vi "getDescription.vi"(8 "error in (no error)":errorcluster, 11 "Xcite in":refnum<class "Xcite.lvclass">) -> (0 "error out":errorcluster, 2 "description":T1={"serial"=0, "type"=65535, "name"="", "wavelenghts_vec"=[], "exclusivity_vec"=[], "intensity_max_vec"=[], "intensity_min_vec"=[]} {"type" items=["XC_120PC"=0, "XC_exacte"=1, "XC_120LED"=2, "XC_110LED"=3, "XC_mini"=4, "XC_XYLIS"=5, "XC_XR210"=6, "XC_LED1"=7, "XC_XT600"=8, "XC_XT900"=9, "Any"=65535]}, 3 "Xcite out":refnum<class "Xcite.lvclass">)   [LabVIEW 2019, in "Xcite.lvclass"]
doc: "Gets the serial number, type and other properties of the XCite device"
uses:
  Xcite.lvclass
  Xcite.lvclass/Xcite.ctl
  etc.xcite/XCite.lvlib
panel:
  out "XCiteType":u16(ring) format="%x" items=["XC_120PC"=0, "XC_exacte"=1, "XC_120LED"=2, "XC_110LED"=3, "XC_mini"=4, "XC_XYLIS"=5, "XC_XR210"=6, "XC_LED1"=7, "XC_XT600"=8, "XC_XT900"=9, "Any"=65535]
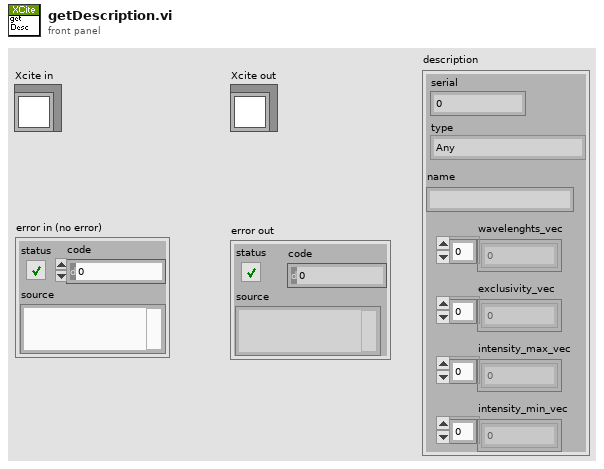
[diagram p1: front panel]
types:
  T1 = cluster{"serial":u32, "type":u16, "name":string, "wavelenghts_vec":u32[], "exclusivity_vec":u32[], "intensity_max_vec":u32[], "intensity_min_vec":u32[]}
  T2 = cluster{"LightSourceName":string, "hDevice":u64, "hCamera":u64, "iNumChannels":i32, "iNumWheels":i32, "dwSystemState":u32, "dwSerialNumber":u32, "dwSystemCaps":u32, "iLastChannelOnWheel":i16[], "XCiteChannels":cluster{"szLedName":string, "iWaveLength":i32, "IBelongToWheelNumber":i32, "iIntensity":i32, "iIntensityMin":i32, "iIntensityMax":i32, "iIntensityStep":i32, "iExtTriggerNum":i32, "iLedTemp":i32, "dwLEDState":u32}[]}
  T3 = cluster{"szLedName":string, "iWaveLength":i32, "IBelongToWheelNumber":i32, "iIntensity":i32, "iIntensityMin":i32, "iIntensityMax":i32, "iIntensityStep":i32, "iExtTriggerNum":i32, "iLedTemp":i32, "dwLEDState":u32}[]
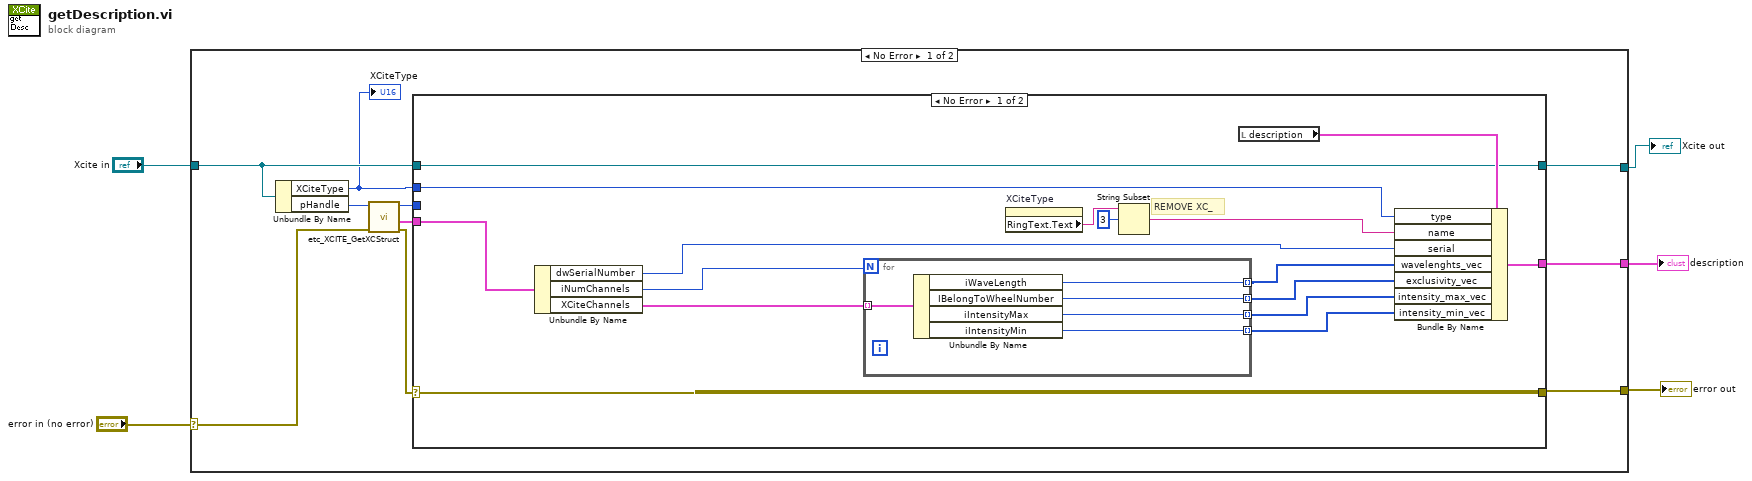
[diagram p0: block diagram]
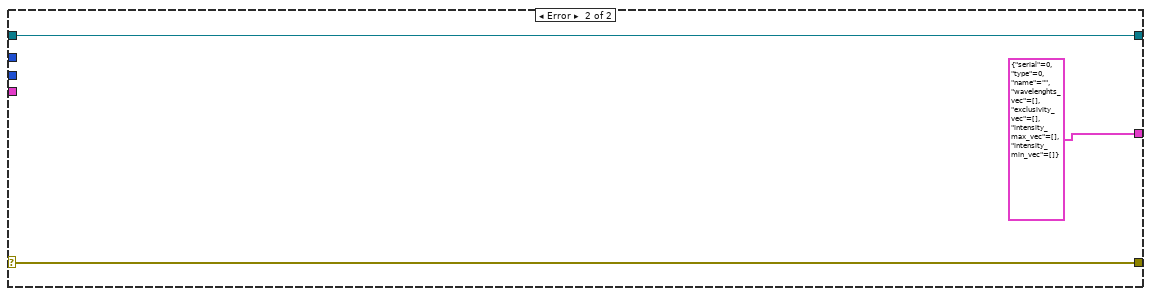
[diagram p2: hidden frame]
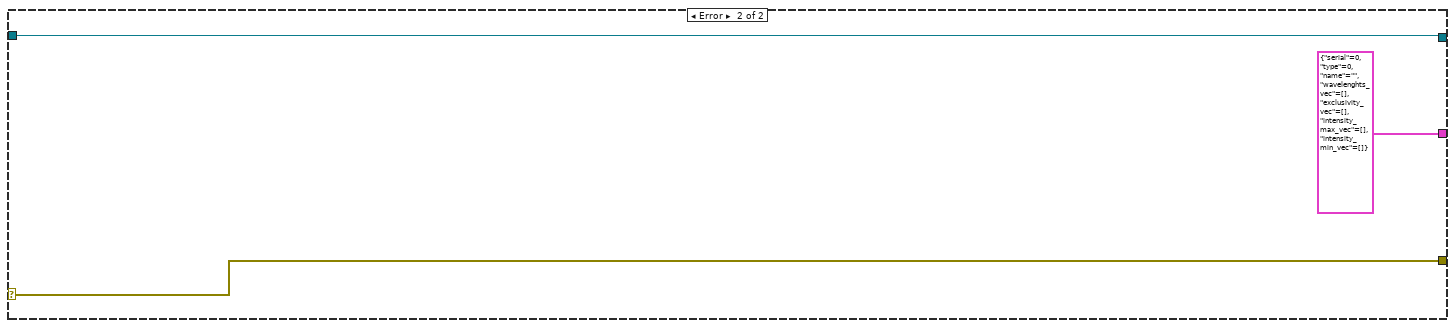
[diagram p3: hidden frame]
diagram:
  n1 = case shown="No Error" "error in (no error)" {
    selector: "error in (no error)" -> [w14 w42]
    tunnel: [w12 w42] -> w4
    tunnel: "Xcite in" -> [w8 w41]
    tunnel: [w9 T1 {"serial"=0, "type"=0, "name"="", "wavelenghts_vec"=[], "exclusivity_vec"=[], "intensity_max_vec"=[], "intensity_min_vec"=[]} ("XCITE_Description")] -> w2
    tunnel: [w7 w41] -> w1
    frame No Error {
      n2 = Unbundle By Name(w8) -> ("XCiteType"=w6:u16, "pHandle"=w15:u64)
      "XCiteType" <- w6
      n3 = call "etc_XCITE_GetXCStruct.vi"("error in (no error)"=w14, "h"=w15) -> ("error out"=w13:errorcluster, "XCiteStructure"=w11:T2, "h out"=w10:u64)  [unwired: 6 in, 1 out]
      n4 = case shown="No Error" w13 {
        selector: w13 -> [w30 w39]
        tunnel: [w30 w39] -> w12
        tunnel: w11 -> [w31 _]
        tunnel: w10 -> [_ _]
        tunnel: w8 -> [w25 w38]
        tunnel: [w26 T1 {"serial"=0, "type"=0, "name"="", "wavelenghts_vec"=[], "exclusivity_vec"=[], "intensity_max_vec"=[], "intensity_min_vec"=[]} ("XCITE_Description")] -> w9
        tunnel: [w25 w38] -> w7
        tunnel: w6 -> [w19 _]
        frame No Error {
          # "REMOVE XC_"
          n5 = Unbundle By Name(w31) -> ("dwSerialNumber"=w20:u32, "iNumChannels"=w28:i32, "XCiteChannels"=w27:T3)
          n6 = for {
            N: w28 -> [_]
            tunnel: w27 -> [w36] mode=indexing
            tunnel: [w35] -> w21 mode=indexing
            tunnel: [w34] -> w22 mode=indexing
            tunnel: [w33] -> w24 mode=indexing
            tunnel: [w32] -> w23 mode=indexing
            n7 = Unbundle By Name(w36) -> ("iWaveLength"=w35:i32, "IBelongToWheelNumber"=w34:i32, "iIntensityMax"=w32:i32, "iIntensityMin"=w33:i32)
          }
          n8 = property on="XCiteType" class="Ring (strict)"() -> ("RingText.Text"=w17:string)  [unwired: 2 in, 2 out]
          n9 = String Subset(string=w17, offset (0)=3) -> (substring=w16:string)  [unwired: 1 in]
          n10 = local read "description"() -> (w29:T1)
          n11 = Bundle By Name(cluster=w29, "type"=w19, "name"=w16, "serial"=w20, "wavelenghts_vec"=w21, "exclusivity_vec"=w22, "intensity_max_vec"=w23, "intensity_min_vec"=w24) -> (w26:T1)
        }
        frame Error {
        }
      }
    }
    frame Error {
    }
  }
  "Xcite out" <- w1
  "error out" <- w4
  "description" <- w2
